vi "Handle KEX Failure.vi"(8 "error in (no error)":errorcluster) -> (0 "error out":errorcluster, 2 "KEX Failure":bool)   [LabVIEW 2017, in "support.lvlib"]
uses:
  support.lvlib
  <vilib>/Utility/error.llb/DialogType.ctl
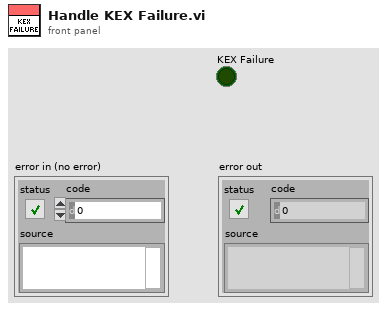
[diagram p1: front panel]
types:
  T1 = typedef "DialogType.ctl" = u16
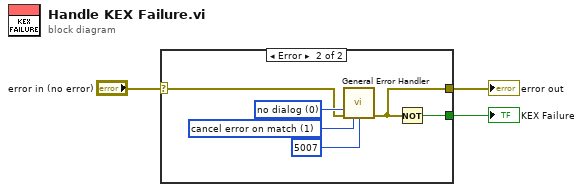
[diagram p0: block diagram]
diagram:
  n1 = case shown="Error" "error in (no error)" {
    selector: "error in (no error)" -> [w4 w7]
    tunnel: [w4 w6] -> w2
    tunnel: [_ w5] -> w1
    frame No Error {
    }
    frame Error {
      w9 = T1 0 items=["no dialog", "OK message", "continue or stop message", "OK message + warnings", "continue/stop + warnings"] ("type of dialog (OK msg:1)")
      w10 = 1 items=["no exception", "cancel error on match", "set error on match"] ("[exception action] (none:0)")
      n2 = call <vilib>:"General Error Handler.vi"("type of dialog (OK msg:1)"=w9, "error in (no error)"=w7, "[exception action] (none:0)"=w10, "[exception code]"=5007 ("specific error code to clear (0: all)")) -> ("error out"=w6:errorcluster)  [unwired: 7 in, 4 out]
      n3 = Not(x=w6) -> (.not. x?=w5:bool)
    }
  }
  "error out" <- w2
  "KEX Failure" <- w1
